vi "Main.vi"(11 "Actor Script Strategy in":refnum<class "Actor Script Strategy.lvclass">) -> ()   [LabVIEW 2021, in "_Create From Template.lvlib" / "Script Strategy.lvlib" / "Actor Script Strategy.lvclass"]
uses:
  Actor Script Strategy.lvclass
  Actor Script Strategy.lvclass/Actor Script Strategy.ctl
  Script Strategy.lvlib
  <vilib>/Utility/EditLVLibs/Edit LVLibs.lvlib
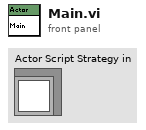
[diagram p1: front panel]
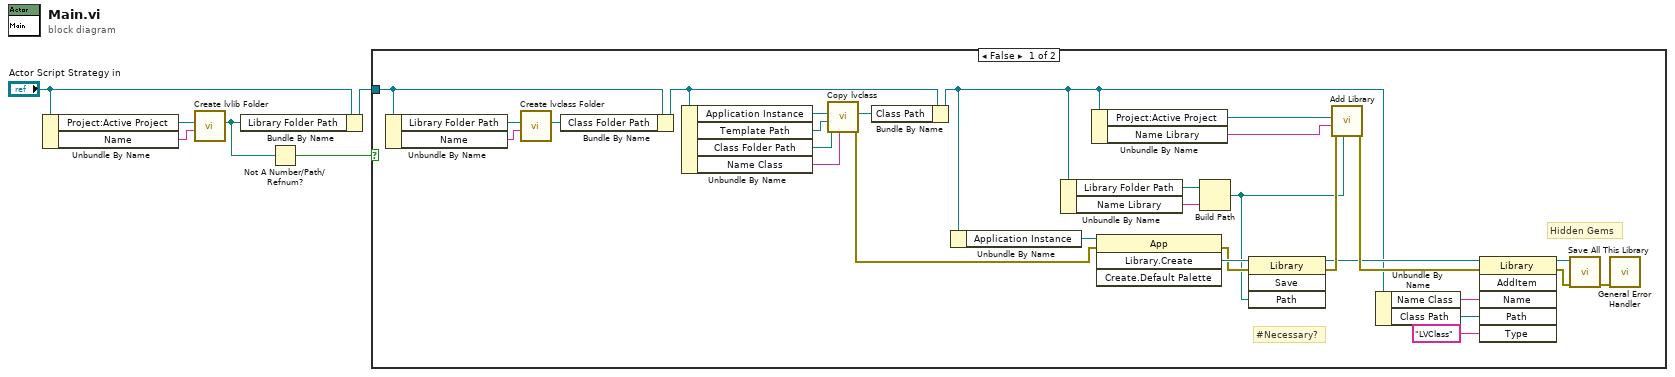
[diagram p0: block diagram]
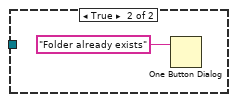
[diagram p2: hidden frame]
diagram:
  n1 = Unbundle By Name("Actor Script Strategy in") -> ("Project:Active Project"=w6:refnum<vi>, "Name"=w5:string)
  n2 = call "Create lvlib Folder.vi"("Name"=w5, "Project:Active Project"=w6) -> ("Library Folder Path"=w2:path)  [unwired: 9 in]
  n3 = Bundle By Name(cluster="Actor Script Strategy in", "Library Folder Path"=w2) -> (w3:refnum<class "Actor Script Strategy.lvclass">)
  n4 = Not A Number/Path/Refnum?(number/path/refnum=w2) -> (NaN/Path/Refnum?=w1:bool)
  n5 = case shown="False" w1 {
    tunnel: w3 -> [w33 _]
    frame False {
      # "#Necessary?"
      # "Hidden Gems"
      n6 = Unbundle By Name(w33) -> ("Library Folder Path"=w32:path, "Name"=w31:string)
      n7 = call "Create lvclass Folder.vi"("Name"=w31, "Library Folder Path"=w32) -> ("Class Folder Path"=w30:path)  [unwired: 9 in]
      n8 = Bundle By Name(cluster=w33, "Class Folder Path"=w30) -> (w24:refnum<class "Actor Script Strategy.lvclass">)
      n9 = Unbundle By Name(w24) -> ("Application Instance"=w29:refnum<vi>, "Template Path"=w27:path, "Class Folder Path"=w26:path, "Name Class"=w25:string)
      n10 = call "Copy lvclass.vi"("Name Class"=w25, "Class Folder Path"=w26, "Template Path"=w27, "Application Instance"=w29) -> ("error out"=w11:errorcluster, "New Library Path"=w28:path)  [unwired: 6 in]
      n11 = Bundle By Name(cluster=w24, "Class Path"=w28) -> (w10:refnum<class "Actor Script Strategy.lvclass">)
      n12 = Unbundle By Name(w10) -> ("Application Instance"=w16:refnum<vi>)
      n13 = Unbundle By Name(w10) -> ("Library Folder Path"=w17:path, "Name Library"=w21:string)
      n14 = Unbundle By Name(w10) -> ("Project:Active Project"=w8:refnum<vi>, "Name Library"=w7:string)
      n15 = invoke class="App" method="Library.Create"(reference=w16, error in=w11) -> (error out=w14:errorcluster, "Create Library"=w15:refnum<vi>)  [unwired: 2 in, 2 out]
      n16 = Build Path(base path=w17, name or relative path=w21) -> (appended path=w9:path)
      n17 = invoke class="Library" method="Save"(reference=w15, error in=w14, "Path"=w9) -> (reference out=w22:refnum<vi>, error out=w34:errorcluster)  [unwired: 1 in, 2 out]
      n18 = call "Add Library.vi"("Library Path"=w9, "error in"=w34, "Name Library"=w7, "Project:Active Project"=w8) -> ("error out"=w35:errorcluster)  [unwired: 7 in]
      n19 = Unbundle By Name(w10) -> ("Name Class"=w19:string, "Class Path"=w20:path)
      n20 = invoke class="Library" method="AddItem"(reference=w22, error in=w35, "Name"=w19, "Path"=w20, "Type"="LVClass") -> (reference out=w18:refnum<vi>, error out=w13:errorcluster)  [unwired: 1 in, 4 out]
      n21 = call <vilib>:"Save All This Library.vi"("error in (no error)"=w13, "Library in"=w18) -> ("error out"=w23:errorcluster)  [unwired: 8 in, 1 out]
      n22 = call <vilib>:"General Error Handler.vi"("error in (no error)"=w23) -> ()  [unwired: 10 in, 5 out]
    }
    frame True {
      n23 = One Button Dialog(message="Folder already exists") -> ()  [unwired: 1 in, 1 out]
    }
  }
